vi "REM IO - Compare ECAT Vars.vi"(8 "Fehler (Eingang, kein Fehler)":errorcluster, 11 "I/O Vars In":T1[](array[typedef]) {"VS ref" format="%.0x"}) -> (0 "Fehler (Ausgang)":errorcluster, 3 "I/O Vars Out":T1[](array[typedef]) {"VS ref" format="%.0x"})   [LabVIEW 2020, in "SEECD Engine.lvlib"]
uses:
  SEECD Engine.lvlib
  Type Defs/REM IO ECAT Slave IOV Cluster.ctl
  <vilib>/NI VeriStand/Custom Device API/Custom Device Item Ref.ctl
  Shared/Type Defs/UDV Data Type.ctl
  Shared/Globals/Property Strings.vi
  <vilib>/NI VeriStand/Custom Device API/Get Item Property (String).vi
  <vilib>/NI VeriStand/Custom Device API/Get Item Property (I32).vi
  Shared/Globals/Error Strings.vi
  <vilib>/NI VeriStand/Custom Device API/Custom Device API.lvlib
  Shared/SEECD Shared.lvlib
  <vilib>/NI VeriStand/Custom Device Tools/Custom Device Utility Library/Custom Device Utility Library.lvlib
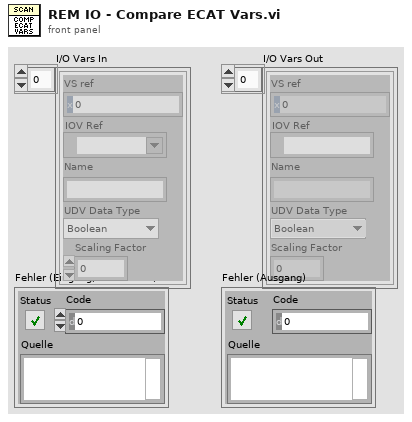
[diagram p1: front panel]
types:
  T1 = typedef "SEECD Engine.lvlib/REM IO ECAT Slave IOV Cluster.ctl" = cluster{"VS ref":T2, "IOV Ref":refnum<k21>, "Name":string, "UDV Data Type":T3, "Scaling Factor":dbl}
  T2 = typedef "Custom Device API.lvlib/Custom Device Item Ref.ctl" = u64
  T3 = typedef "SEECD Shared.lvlib/UDV Data Type.ctl" = enum16{"Boolean", "Fixed Point", "Int8", "Int16", "Int32", "Int64", "U32 Bit Field", "UInt8", "UInt16", "UInt32", "UInt64", "Other", "DBL", "SGL"}
  T4 = typedef "Custom Device API.lvlib/Custom Device Item Info.ctl" = cluster{"Name":string, "Is Channel":bool, "GUID":string, "Is Waveform":bool}
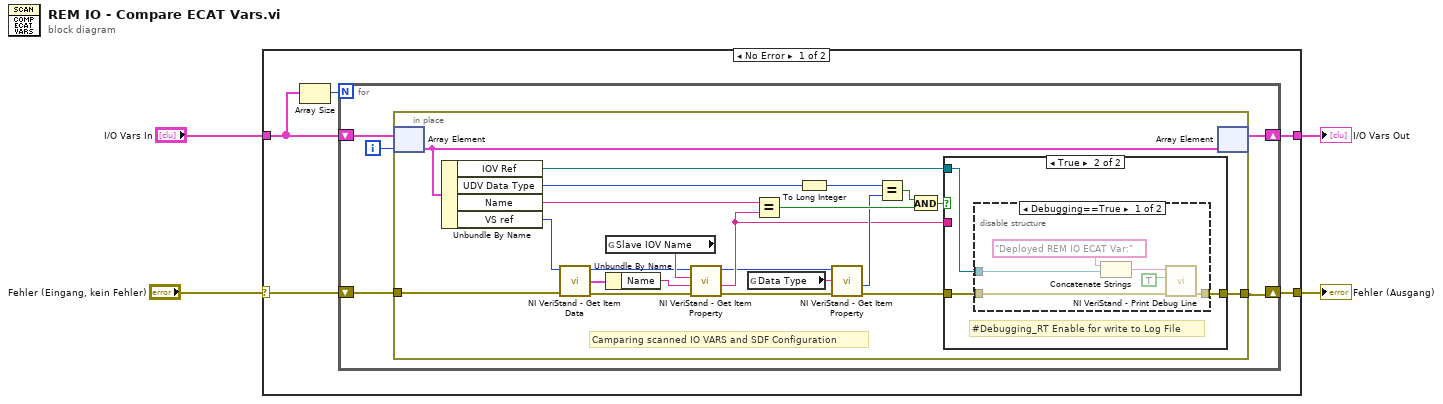
[diagram p0: block diagram]
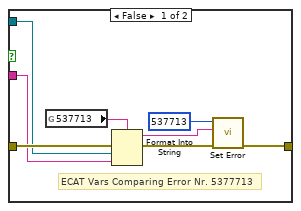
[diagram p2: hidden frame]
diagram:
  n1 = case shown="No Error" "Fehler (Eingang, kein Fehler)" {
    selector: "Fehler (Eingang, kein Fehler)" -> [w8 w56]
    tunnel: [w5 w55] -> w1
    tunnel: [w7 w56] -> w4
    tunnel: "I/O Vars In" -> [w6 w55]
    frame No Error {
      n2 = Array Size(array=w6) -> (size(s)=w9:i32)
      n3 = for {
        N: w9 -> [_]
        shift-right: [w12] -> w7
        shift-left: w8 -> [w13]
        shift-right: [w10] -> w5
        shift-left: w6 -> [w11]
        i -> [w14]
        n4 = in-place {
          in-place-border: w13 -> [w35]
          in-place-border: [w30] -> w12
          # "Camparing scanned IO VARS and SDF Configuration"
          n5 = in-place-array #1(w11, w14) -> (w26:T1)
          n6 = Unbundle By Name(w26) -> ("IOV Ref"=w28:refnum<k21>, "UDV Data Type"=w29:T3, "Name"=w25:string, "VS ref"=w27:T2)
          n7 = call <vilib>:"NI VeriStand - Get Item Data.vi"("error in (no error)"=w35, "Item Ref in"=w27) -> ("error out"=w18:errorcluster, "Item Info"=w20:T4, "Item Ref out"=w16:T2)  [unwired: 6 in, 1 out]
          n8 = global read "Property Strings.vi" "Slave IOV Name"() -> (w22:string)
          n9 = Unbundle By Name(w20) -> ("Name"=w19:string)
          n10 = call-poly <vilib>:"NI VeriStand - Get Item Property.vi"("error in (no error)"=w18, "Default Value"=w19, "Property Name"=w22, "Item Ref in"=w16) -> ("error out"=w17:errorcluster, "Value"=w21:string, "Item Ref out"=w15:T2)  [unwired: 4 in, 1 out]
          n11 = global read "Property Strings.vi" "Data Type"() -> (w36:string)
          n12 = Equal?(x=w25, y=w21) -> (x = y?=w33:bool)
          n13 = To Long Integer(number=w29) -> (32bit integer=w23:i32)
          n14 = call-poly <vilib>:"NI VeriStand - Get Item Property.vi"("error in (no error)"=w17, "Property Name"=w36, "Item Ref in"=w15) -> ("error out"=w31:errorcluster, "Value"=w24:i32)  [unwired: 5 in, 2 out]
          n15 = Equal?(x=w23, y=w24) -> (x = y?=w34:bool)
          n16 = And(x=w34, y=w33) -> (x .and. y?=w32:bool)
          n17 = case shown="True" w32 {
            tunnel: w31 -> [w40 w47]
            tunnel: [w39 w46] -> w30
            tunnel: w28 -> [w38 w45]
            tunnel: w21 -> [w37 _]
            frame False {
              # "ECAT Vars Comparing Error Nr. 5377713"
              n18 = global read "Error Strings.vi" "537713"() -> (w41:string)
              n19 = Format Into String(format string=w41, error in=w40, w38, w37) -> (resulting string=w43:string, error out=w42:errorcluster)  [unwired: 1 in]
              n20 = call "Set Error.vi"("error in (no error)"=w42, "Message"=w43, "Code"=537713 ("error code (0)")) -> ("error out"=w39:errorcluster)  [unwired: 8 in]
            }
            frame True {
              # "#Debugging_RT Enable for write to Log File"
              n21 = disable-structure shown="Debugging==True" {
                disable-tunnel: w47 -> [w53 w54]
                disable-tunnel: [w52 w54] -> w46
                disable-tunnel: w45 -> [w49 _]
                frame condition #0 {
                  n22 = Concatenate Strings("Deployed REM IO ECAT Var:", w49) -> (w51:string)
                  n23 = call <vilib>:"NI VeriStand - Print Debug Line.vi"("error in (no error)"=w53, "Add to log file? (F)"=TRUE, "Message"=w51) -> ("error out"=w52:errorcluster)  [unwired: 8 in]
                }
                frame condition #1 (active) {
                }
              }
            }
          }
          n24 = in-place-array #1(w26) -> (w10:T1[])  [unwired: 1 out]
        }
      }
    }
    frame Error {
    }
  }
  "I/O Vars Out" <- w1
  "Fehler (Ausgang)" <- w4
